vi "binario.vi"(8 "error in (no error)":errorcluster, 10 "signal out":waveform(dbl), 11 "BINARIO in":refnum<class "BINARIO.lvclass">) -> (0 "error out":errorcluster, 3 "BINARIO out":refnum<class "BINARIO.lvclass">)   [LabVIEW 2020, in "BINARIO.lvlib" / "BINARIO.lvclass"]
uses:
  BINARIO.lvclass
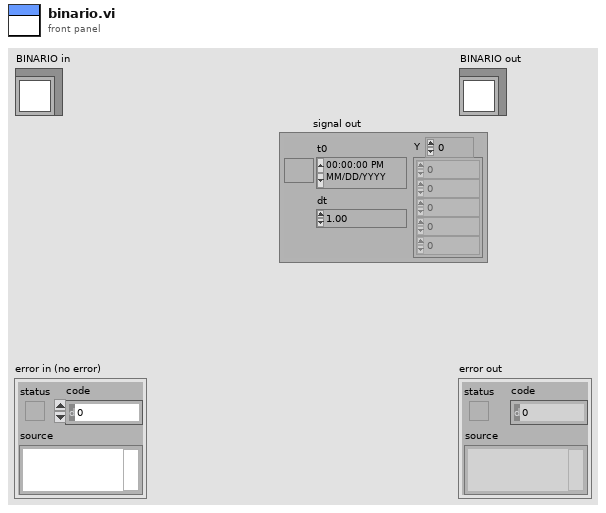
[diagram p1: front panel]
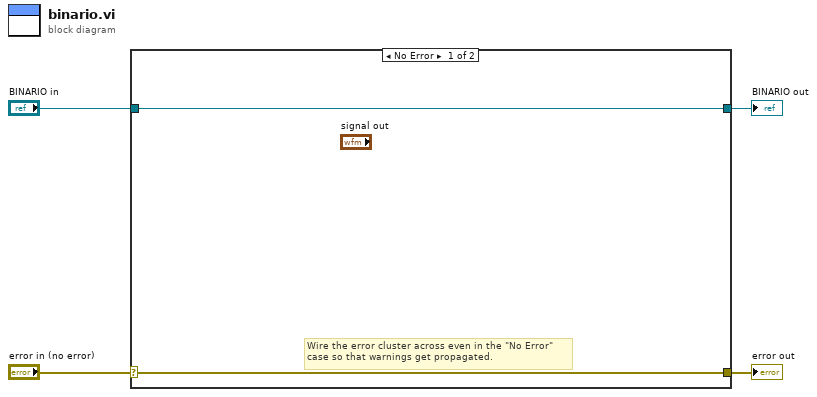
[diagram p0: block diagram]
diagram:
  n1 = case shown="No Error" "error in (no error)" {
    selector: "error in (no error)" -> [w5 w8]
    tunnel: [w5 w8] -> w3
    tunnel: [w6 w7] -> w1
    tunnel: "BINARIO in" -> [w6 w7]
    frame No Error {
      # "Wire the error cluster across even in the \"No Error\"\ncase so that warnings get propagated."
    }
    frame Error {
    }
  }
  "error out" <- w3
  "BINARIO out" <- w1
